vi "效率计算_sub.vi"(8 "输出电流":dbl format="%.3g", 9 "输出电压":dbl format="%.3g", 10 "输入电流":dbl format="%.3g", 11 "输入电压":dbl format="%.3g") -> (0 "效率":dbl format="%.1f%%")   [LabVIEW 2012]
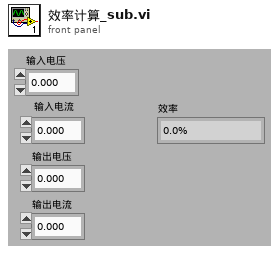
[diagram p1: front panel]
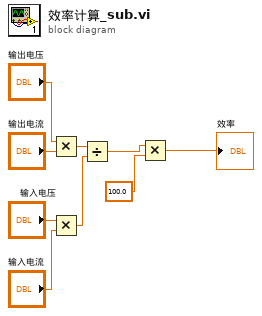
[diagram p0: block diagram]
diagram:
  n1 = Multiply(x="输出电压", y="输出电流") -> (x*y=w4:dbl)
  n2 = Multiply(x="输入电压", y="输入电流") -> (x*y=w5:dbl)
  n3 = Divide(x=w4, y=w5) -> (x/y=w3:dbl)
  n4 = Multiply(x=w3, y=100.0) -> (x*y=→"效率":dbl)
